vi "Parse_FRH_Type_String.vi"(1 "String In":string, 2 "All IDs?":bool=TRUE, 3 "IDs In":i32[](array[numeric])) -> (14 "Parsed Cluster Out":T1(array[cluster]), 15 "String 1 Out":string[](array[string]), 16 "String 2 Out":string[](array[string]), 17 "IDs Out":i32[](array[numeric]))   [LabVIEW 2020]
doc: "Returns ID, String 1 and String 2 for String In. String In must be in FRH? reply format (ID1 = String1 TAB String2 Space LF ID2 = String 3 TAB String 4 Space LF end of help LF). If All IDs? is FALSE, parsed strings are returned for IDs In only."
panel:
  # "Returns ID, String 1 and String 2 for String In. String In must be in FRH? reply format. If \"All IDs?\" is FALSE, parsed strings are returned for IDs In only."
  # "If not:"
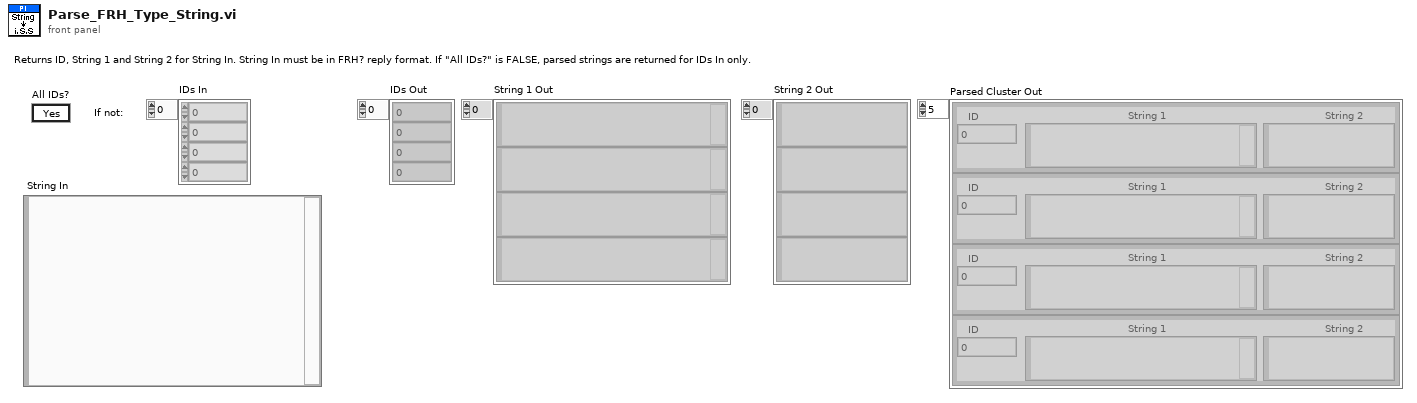
[diagram p1: front panel]
types:
  T1 = cluster{"ID":i32, "String 1":string, "String 2":string}[]
  T2 = cluster{"ResultID":i32, "Meaning":string, "Unit":string}[]
  T3 = cluster{"ID":i32, "String 1":string, "String 2":string}
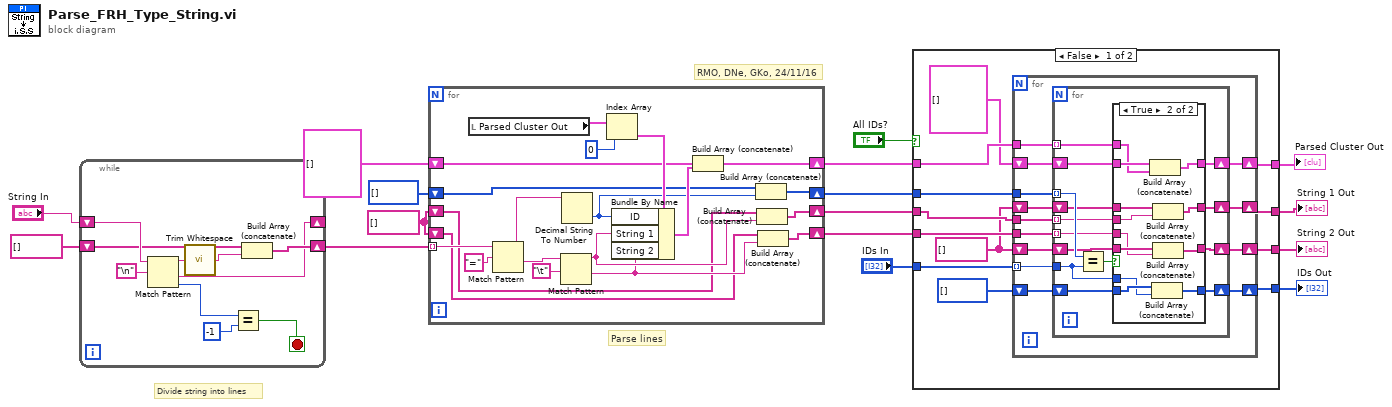
[diagram p0: block diagram]
diagram:
  w13 = string[] []
  # "Parse lines"
  # "Divide string into lines"
  # "RMO, DNe, GKo, 24/11/16"
  n1 = while {
    shift-right: [w21] -> _
    shift-left: "String In" -> [w26]
    shift-right: [w22] -> w12
    shift-left: string[] [] -> [w23]
    stop <- w20 stop-if-true
    n2 = Match Pattern(string=w26, regular expression="\n") -> (before substring=w18:string, after substring=w21:string, offset past match=w24:i32)  [unwired: 2 out]
    n3 = call "Trim Whitespace.vi"("string"=w18) -> ("trimmed string"=w17:string)  [unwired: 1 in]
    n4 = Equal?(x=w24, y=-1) -> (x = y?=w20:bool)
    n5 = Build Array (concatenate)(w23, w17) -> (w22:string[])
  }
  n6 = for {
    tunnel: w12 -> [w46] mode=indexing
    shift-right: [w38] -> w7
    shift-left: T2 [] -> [w36]
    shift-right: [w33] -> w9
    shift-left: i32[] [] -> [w29]
    shift-right: [w35] -> w5
    shift-left: w13 -> [w28]
    shift-right: [w34] -> w4
    shift-left: w13 -> [w27]
    n7 = local read "Parsed Cluster Out"() -> (w41:T1)
    n8 = Match Pattern(string=w46, regular expression="=") -> (before substring=w42:string, after substring=w43:string)  [unwired: 3 out]
    n9 = Match Pattern(string=w43, regular expression="\t") -> (before substring=w31:string, after substring=w30:string)  [unwired: 3 out]
    n10 = Decimal String To Number(string=w42) -> (number=w32:i32)  [unwired: 3 out]
    n11 = Index Array(array=w41, index=0) -> (element=w39:T3)
    n12 = Bundle By Name(cluster=w39, "ID"=w32, "String 1"=w31, "String 2"=w30) -> (w37:T3)
    n13 = Build Array (concatenate)(w36, w37) -> (w38:T1)
    n14 = Build Array (concatenate)(w29, w32) -> (w33:i32[])
    n15 = Build Array (concatenate)(w28, w31) -> (w35:string[])
    n16 = Build Array (concatenate)(w27, w30) -> (w34:string[])
  }
  n17 = case shown="False" "All IDs?" {
    tunnel: w9 -> [w57 w105]
    tunnel: [w55 w105] -> w8
    tunnel: w7 -> [w51 w104]
    tunnel: [w56 w104] -> w6
    tunnel: w5 -> [w50 w103]
    tunnel: w4 -> [w49 w102]
    tunnel: [w53 w103] -> w3
    tunnel: [w54 w102] -> w2
    tunnel: "IDs In" -> [w58 _]
    frame False {
      w48 = string[] []
      n18 = for {
        tunnel: w58 -> [w71] mode=indexing
        shift-right: [w69] -> w56
        shift-left: T2 [] -> [w68]
        shift-right: [w67] -> w55
        shift-left: i32[] [] -> [w64]
        shift-right: [w65] -> w53
        shift-left: w48 -> [w62]
        shift-right: [w66] -> w54
        shift-left: w48 -> [w63]
        tunnel: w57 -> [w70]
        tunnel: w51 -> [w61]
        tunnel: w50 -> [w60]
        tunnel: w49 -> [w59]
        n19 = for {
          tunnel: w70 -> [w85] mode=indexing
          tunnel: w71 -> [w81]
          shift-right: [w83] -> w69
          shift-left: w68 -> [w82]
          shift-right: [w80] -> w67
          shift-left: w64 -> [w77]
          shift-right: [w78] -> w65
          shift-left: w62 -> [w75]
          shift-right: [w79] -> w66
          shift-left: w63 -> [w76]
          tunnel: w61 -> [w74] mode=indexing
          tunnel: w60 -> [w73] mode=indexing
          tunnel: w59 -> [w72] mode=indexing
          n20 = Equal?(x=w85, y=w81) -> (x = y?=w84:bool)
          n21 = case shown="True" w84 {
            tunnel: [w89 w100] -> w83
            tunnel: w82 -> [w89 w101]
            tunnel: w81 -> [_ w93]
            tunnel: [w88 w99] -> w80
            tunnel: [w87 w98] -> w79
            tunnel: [w86 w97] -> w78
            tunnel: w77 -> [w88 w96]
            tunnel: w76 -> [w87 w95]
            tunnel: w75 -> [w86 w94]
            tunnel: w74 -> [_ w92]
            tunnel: w73 -> [_ w91]
            tunnel: w72 -> [_ w90]
            frame False {
            }
            frame True {
              n22 = Build Array (concatenate)(w101, w92) -> (w100:T2)
              n23 = Build Array (concatenate)(w96, w93) -> (w99:i32[])
              n24 = Build Array (concatenate)(w94, w91) -> (w97:string[])
              n25 = Build Array (concatenate)(w95, w90) -> (w98:string[])
            }
          }
        }
      }
    }
    frame True {
    }
  }
  "String 1 Out" <- w3
  "String 2 Out" <- w2
  "Parsed Cluster Out" <- w6
  "IDs Out" <- w8
